vi "2DGaussianFit.vi"(3 "error in (no error)":errorcluster, 4 "Nb Pts X&Y":i32=30, 5 "Input Image Array":u16[][](array[numeric])) -> (0 "error out":errorcluster, 1 "Scanned Image":u16[][](graph), 2 "Best Fit":dbl[](array[numeric]) format="%.2f")   [LabVIEW 2015]
uses:
  <vilib>/gmath/NumericalOptimization/Nonlinear Curve Fit LM.vi
  <vilib>/gmath/NI_Gmath.lvlib
panel:
  out "transposed array":i32[][](array[numeric])
  out "Parameter Names":string[](array[string])=["Xposition", "Xwidth", "Yposition", "Ywidth", "Amplitude"]
  # "X"
  # "Y"
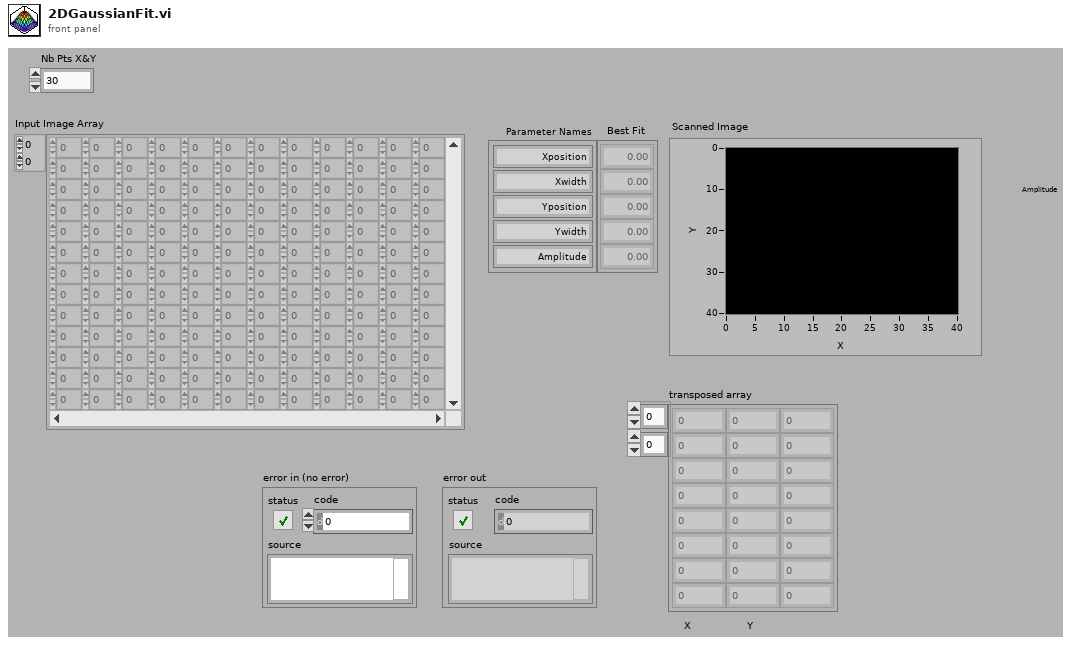
[diagram p1: front panel]
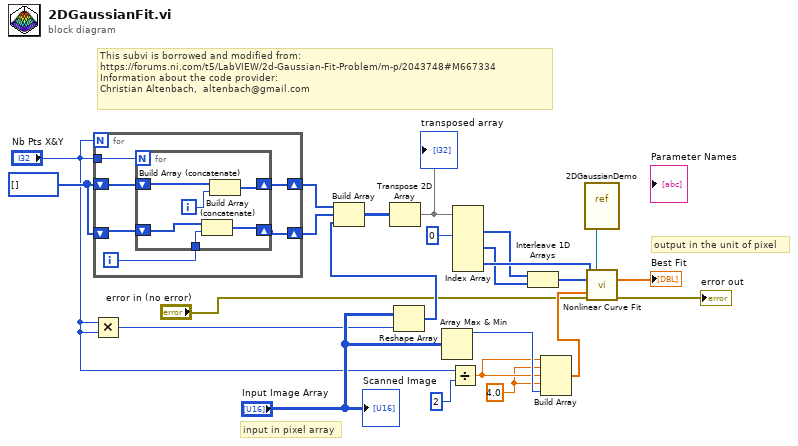
[diagram p0: block diagram]
diagram:
  w4 = 4.0 ("element")
  w16 = i32[] []
  # "This subvi is borrowed and modified from:  \nhttps://forums.ni.com/t5/LabVIEW/2d-Gaussian-Fit-Problem/m-p/2043748#M667334\nInformation about the code provider:\nChristian Altenbach,  altenbach@gmail.com"
  # "input in pixel array"
  # "output in the unit of pixel"
  n1 = Multiply(x="Nb Pts X&Y", y="Nb Pts X&Y") -> (x*y=w9:i32)
  n2 = for {
    N: "Nb Pts X&Y" -> [_]
    tunnel: "Nb Pts X&Y" -> [w29]
    shift-right: [w27] -> w15
    shift-left: w16 -> [w28]
    shift-right: [w25] -> w14
    shift-left: w16 -> [w24]
    i -> [w26]
    n3 = for {
      N: w29 -> [_]
      shift-right: [w34] -> w27
      shift-left: w28 -> [w33]
      tunnel: w26 -> [w32]
      shift-right: [w31] -> w25
      shift-left: w24 -> [w30]
      i -> [w35]
      n4 = Build Array (concatenate)(w30, w32) -> (w31:i32[])
      n5 = Build Array (concatenate)(w33, w35) -> (w34:i32[])
    }
  }
  n6 = Reshape Array("Input Image Array", w9) -> (w13:u16[])
  n7 = Build Array(w15, w14, w13) -> (w12:i32[][])
  n8 = Transpose 2D Array(2D array=w12) -> (transposed array=w17:i32[][])
  "transposed array" <- w17
  n9 = Array Max & Min(array="Input Image Array") -> (max value=w8:u16)  [unwired: 3 out]
  n10 = Divide(x="Nb Pts X&Y", y=2) -> (x/y=w5:dbl)
  n11 = Index Array(array=w17, index (col) #1=0 ("disabled index (col)")) -> (element #1=w3:i32[], element #2=w2:i32[], element #3=w21:i32[])  [unwired: 5 in]
  n12 = Interleave 1D Arrays(w3, w2) -> (w20:i32[])
  n13 = Build Array(w5, w4, w5, w4, w8) -> (w19:dbl[])
  n14 = vi-ref "2DGaussianDemo.vi"() -> (w23:refnum<vi>)
  n15 = call-poly <vilib>:"Nonlinear Curve Fit.vi"("Y"=w21, "f(x,a)"=w23, "X"=w20, "initial parameters"=w19, "error in (no error)"="error in (no error)") -> ("best fit parameters"=→"Best Fit":dbl[], "error out"=→"error out":errorcluster)  [unwired: 5 in, 4 out]
  "Scanned Image" <- "Input Image Array"
